vi "StringCaseString.vi"(5 "selector string":string) -> (1 "Default":bool, 4 "case":string)   [LabVIEW 2014, in "Raspberry Pi Compatible Compiler for LabVIEW.lvlib" / "CaseStructure.lvclass"]
uses:
  CaseStructure.lvclass
  Python/Parsing/ListTypesTD.ctl
  <vilib>/regexp/Match Regular Expression.xnode
  Python/Parsing/Python Functions.lvlib
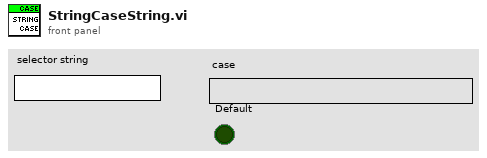
[diagram p1: front panel]
types:
  T1 = typedef "Raspberry Pi Compatible Compiler for LabVIEW.lvlib/Python Functions.lvlib/ListTypesTD.ctl" = enum16{"list", "tuple", "parameter list", "output list", "return values"}
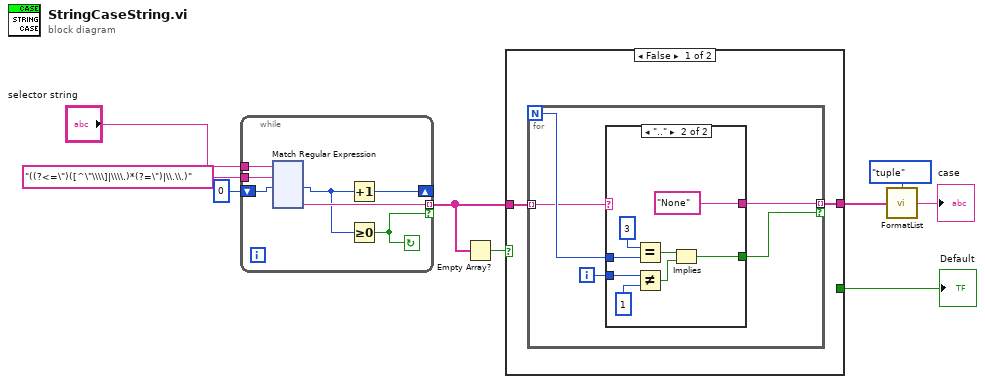
[diagram p0: block diagram]
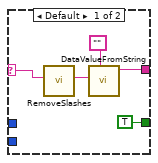
[diagram p2: hidden frame]
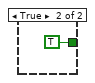
[diagram p3: hidden frame]
diagram:
  n1 = while {
    tunnel: "selector string" -> [w16]
    tunnel: "((?<=\")([^\"\\\\]|\\\\.)*(?=\")|\\.\\.)" ("regular expression") -> [w15]
    tunnel: [w13] -> w1 mode=indexing if=w12
    shift-right: [w10] -> _
    shift-left: 0 -> [w14]
    stop <- w12 continue-if-true
    n2 = xnode "Match Regular Expression"("input string"=w16, "regular expression"=w15, "offset (0)"=w14) -> ("offset past match"=w11:i32, "submatch 1"=w13:string)  [unwired: 3 in, 4 out]
    n3 = Increment(x=w11) -> (x+1=w10:i32)
    n4 = Greater Or Equal To 0?(x=w11) -> (x >= 0?=w12:bool)
  }
  n5 = Empty Array?(array=w1) -> (empty?=w2:bool)
  n6 = case shown="False" w2 {
    tunnel: w1 -> [w131 _]
    tunnel: [w130 _] -> w5
    tunnel: [_ TRUE] -> w4
    frame False {
      n7 = for {
        N -> [w136]
        tunnel: w131 -> [w135] mode=indexing
        tunnel: [w134] -> w130 mode=indexing if=w132
        i -> [w133]
        n8 = case shown="\"..\"" w135 {
          selector: w135 -> [w139 _]
          tunnel: [w141 "None"] -> w134
          tunnel: w133 -> [_ w148]
          tunnel: w136 -> [_ w146]
          tunnel: [TRUE w144] -> w132
          frame Default {
            n9 = call "RemoveSlashes.vi"("slashed string"=w139) -> ("unslashed"=w138:string)  [unwired: 10 in]
            n10 = call "DataValueFromString.vi"("Type"="", "value"=w138) -> ("value"=w141:string)  [unwired: 7 in]
          }
          frame ".." {
            n11 = Equal?(x=3, y=w146) -> (x = y?=w143:bool)
            n12 = Not Equal?(x=w148, y=1) -> (x != y?=w142:bool)
            n13 = Implies(1:w142, 2:w143) -> (0:w144:bool)
          }
        }
      }
    }
    frame True {
    }
  }
  "Default" <- w4
  n14 = call "FormatList.vi"("values"=w5, "type"=ListTypesTD."tuple") -> ("python object"=→"case":string)
